vi "Toggle Value.vi"(8 "error in (no error)":errorcluster, 10 "Index":i32, 11 "MCListbox with Checkboxes in":refnum<class "MCListbox with Checkboxes.lvclass">) -> (0 "error out":errorcluster, 3 "MCListbox with Checkboxes out":refnum<class "MCListbox with Checkboxes.lvclass">)   [LabVIEW 2016, in "MCListbox with Checkboxes.lvclass"]
uses:
  MCListbox with Checkboxes.lvclass
  MCListbox with Checkboxes.lvclass/MCListbox with Checkboxes.ctl
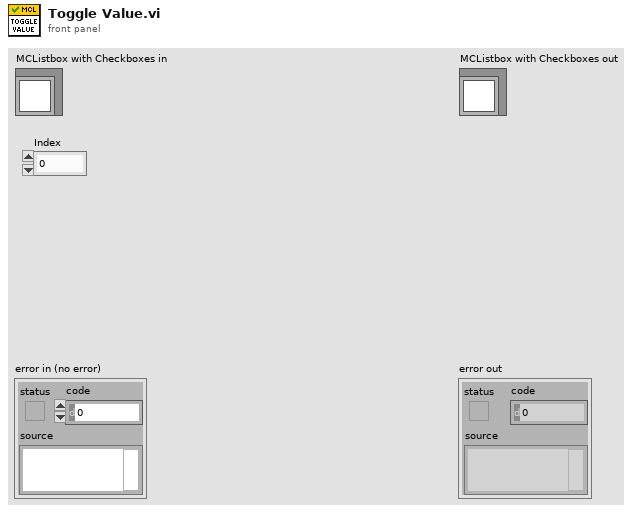
[diagram p1: front panel]
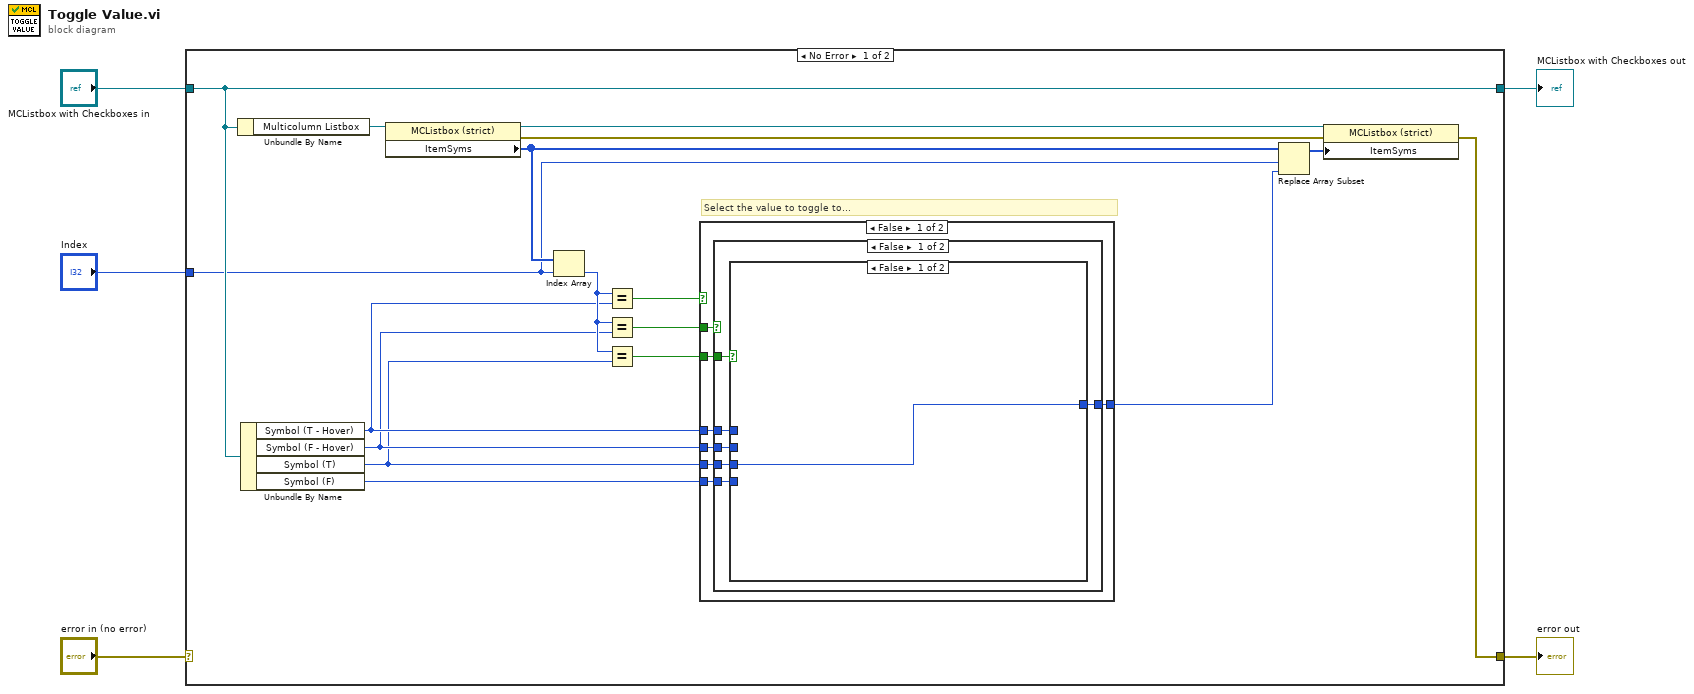
[diagram p0: block diagram]
diagram:
  n1 = case shown="No Error" "error in (no error)" {
    selector: "error in (no error)" -> [_ w41]
    tunnel: [w8 w41] -> w4
    tunnel: [w21 w40] -> w2
    tunnel: "MCListbox with Checkboxes in" -> [w21 w40]
    tunnel: "Index" -> [w6 _]
    frame No Error {
      # "Select the value to toggle to..."
      n2 = Unbundle By Name(w21) -> ("Multicolumn Listbox"=w22:refnum<vi>)
      n3 = Unbundle By Name(w21) -> ("Symbol (T - Hover)"=w16:i32, "Symbol (F - Hover)"=w15:i32, "Symbol (T)"=w14:i32, "Symbol (F)"=w13:i32)
      n4 = property class="MCListbox (strict)"(reference=w22) -> (reference out=w9:refnum<vi>, error out=w10:errorcluster, "ItemSyms"=w12:i32[])  [unwired: 1 in]
      n5 = Index Array(array=w12, index=w6) -> (element=w20:i32)
      n6 = Equal?(x=w20, y=w16) -> (x = y?=w19:bool)
      n7 = Equal?(x=w20, y=w15) -> (x = y?=w18:bool)
      n8 = Equal?(x=w20, y=w14) -> (x = y?=w17:bool)
      n9 = case shown="False" w19 {
        tunnel: w18 -> [w29 _]
        tunnel: w17 -> [w28 _]
        tunnel: w16 -> [w27 _]
        tunnel: w15 -> [w26 w39]
        tunnel: w14 -> [w25 _]
        tunnel: w13 -> [w24 _]
        tunnel: [w23 w39] -> w7
        frame False {
          n10 = case shown="False" w29 {
            tunnel: w28 -> [w35 _]
            tunnel: w27 -> [w34 w38]
            tunnel: w26 -> [w33 _]
            tunnel: w25 -> [w32 _]
            tunnel: w24 -> [w31 _]
            tunnel: [w30 w38] -> w23
            frame False {
              n11 = case shown="False" w35 {
                tunnel: w34 -> [_ _]
                tunnel: w33 -> [_ _]
                tunnel: w32 -> [w36 _]
                tunnel: w31 -> [_ w37]
                tunnel: [w36 w37] -> w30
                frame False {
                }
                frame True {
                }
              }
            }
            frame True {
            }
          }
        }
        frame True {
        }
      }
      n12 = Replace Array Subset(array=w12, new element=w7, index=w6) -> (w11:i32[])
      n13 = property class="MCListbox (strict)"(reference=w9, error in=w10, "ItemSyms"=w11) -> (error out=w8:errorcluster)  [unwired: 1 out]
    }
    frame Error {
    }
  }
  "error out" <- w4
  "MCListbox with Checkboxes out" <- w2
